vi "get_Value_from_Key-ValueClusterArray.vi"(8 "error in (no error)":errorcluster) -> (0 "error out":errorcluster)   [LabVIEW 2015]
doc: "Use this template to build a VI to use as a subVI."
panel:
  in  "key":string
  in  "Key-Value Array":cluster{"value":string}[][](array[cluster])=[[{"value"="Calibrator"}, {"value"="COM12"}], [{"value"="DMM"}, {"value"="COM2"}], [{"value"="Device_names"}, {"value"="Dev1"}], [{"value"="StationID"}, {"value"="TSModisEdge"}], [{"value"="Fixture_SN"}, {"value"="ModisEdgeScopeFixture1"}], [{"value"="AlwaysPrint"}, {"value"="False"}], [{"value"="TestReportPath"}, {"value"="C:\\Snap-On\\ModisEdge_Scope\\"}], [{"value"="ManufactDate"}, {"value"="03-17-2015"}], [{"value"="ManufactLocation"}, {"value"="NeoTech"}], [{"value"="PcbAssemblyNum"}, {"value"="EAP0226L50A"}], [{"value"="PcbRevision"}, {"value"="B"}], [{"value"="LastCalLocation"}, {"value"="NeoTech"}], [{"value"="Delay(s)"}, {"value"="3"}]]
  out "value":string
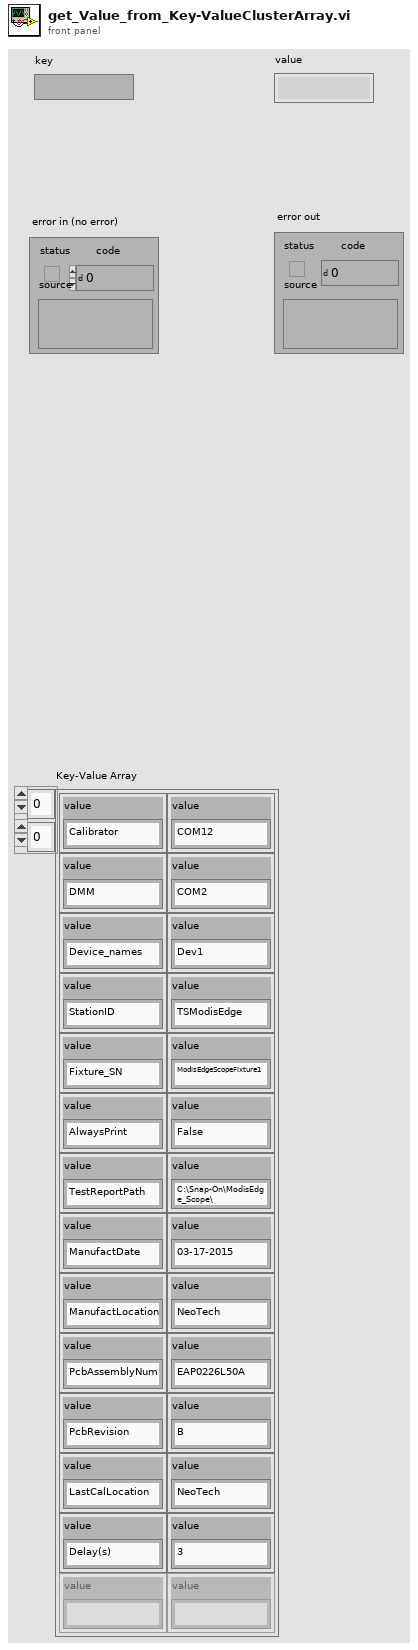
[diagram p1: front panel]
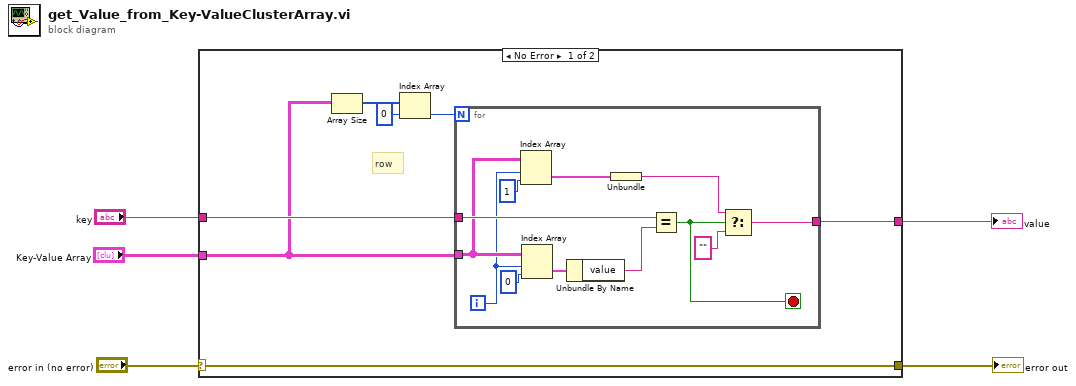
[diagram p0: block diagram]
diagram:
  n1 = case shown="No Error" "error in (no error)" {
    selector: "error in (no error)" -> [w6 w25]
    tunnel: "key" -> [w9 _]
    tunnel: "Key-Value Array" -> [w8 _]
    tunnel: [w7 _] -> w2
    tunnel: [w6 w25] -> w1
    frame No Error {
      # "row"
      n2 = Array Size(array=w8) -> (size(s)=w12:i32[])
      n3 = Index Array(array=w12, index=0) -> (element=w10:i32)
      n4 = for {
        N: w10 -> [_]
        tunnel: w9 -> [w22]
        tunnel: w8 -> [w20]
        tunnel: [w14] -> w7
        i -> [w19]
        stop <- w13 stop-if-true
        n5 = Index Array(array=w20, index (row)=w19, index (col)=1 ("disabled index (col)")) -> (element=w17:cluster{"value":string})
        n6 = Index Array(array=w20, index (row)=w19, index (col)=0 ("disabled index (col)")) -> (element=w23:cluster{"value":string})
        n7 = Unbundle By Name(w23) -> ("value"=w21:string)
        n8 = Unbundle(w17) -> ("value"=w16:string)
        n9 = Equal?(x=w22, y=w21) -> (x = y?=w13:bool)
        n10 = Select(t=w16, s=w13, f="") -> (s? t:f=w14:string)
      }
    }
    frame Error {
    }
  }
  "error out" <- w1
  "value" <- w2
